vi "init.vi"(8 "error in":errorcluster, 10 "TBM module configuration in":refnum<class "TBM module configuration.lvclass">, 11 "shared memory module runtime":refnum<class "Shared Memory Runtime.lvclass">) -> (0 "error out":errorcluster, 1 "data allocations":T1, 2 "execution settings":T4, 3 "shared memory module runtime out":refnum<class "Shared Memory Runtime.lvclass">)   [LabVIEW 2013, in "Shared Memory Runtime.lvclass"]
doc: "Provides an interface for initializing a module at runtime. While this interface performs no operations, a child should provide an override which may open any necessary references or sessions, allocate necessary memory, and perform any final configuration validataion before providing the full configuration <b>execution data</b> to the calling process.Copyright 2016 National Instruments Corporation\n\nLicensed under the Apache License, Version 2.0 (the \"License\"); you may not use this file except in compliance with the License. You may obtain a copy of the License at http://www.apache.org/licenses/LICENSE-2.0\nUnless required by applicable law or agreed to in writing, software distributed under the License is distributed on an \"AS IS\" BASIS, WITHOUT WARRANTIES OR CONDITIONS OF ANY KIND, either express or implied. See the License for the specific language governing permissions and limitations under the License."
uses:
  Shared Memory Runtime.lvclass
  <vilib>/NI/Tag Bus Module Framework/module configuration/TBM module configuration.lvclass
  <vilib>/NI/Tag Bus Module Framework/runtime/execution settings.ctl
  <vilib>/NI/Tag Bus Module Framework/channel/data tables.ctl
  <vilib>/NI/Tag Bus/dictionary/data dictionary.lvclass
  <vilib>/NI/Tag Bus/dictionary table pair.ctl
  <vilib>/NI/Tag Bus/table/data table.ctl
  configuration/Shared Memory Configuration.lvclass
  configuration/Shared Memory Configuration.lvclass/Shared Memory Configuration.ctl
  configuration/Read lines.vi
  configuration/read read directory.vi
  configuration/read write directory.vi
  <vilib>/NI/Tag Bus Module Framework/channel/TBM channel.lvclass
  <vilib>/NI/Tag Bus Module Framework/runtime/TBM module execution interface.lvclass
  <vilib>/NI/Tag Bus/tag bus.lvlib
  <vilib>/NI/Tag Bus/table/data table.lvlib
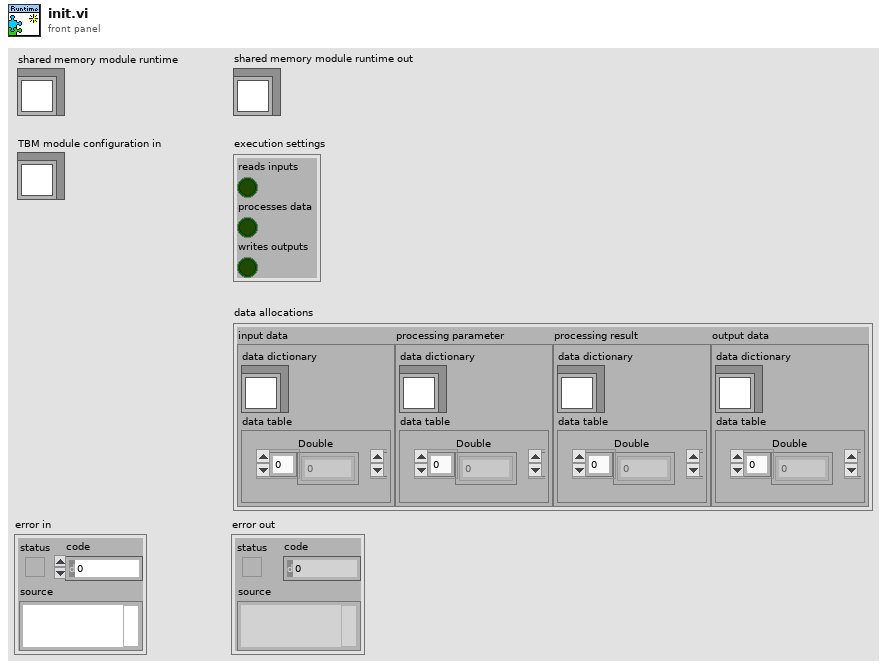
[diagram p1: front panel]
types:
  T1 = typedef "TBM channel.lvclass/data tables.ctl" = cluster{"input data":T2, "processing parameter":T2, "processing result":T2, "output data":T2}
  T2 = typedef "tag bus.lvlib/dictionary table pair.ctl" = cluster{"data dictionary":refnum<class "data dictionary.lvclass">, "data table":T3}
  T3 = typedef "tag bus.lvlib/data table.lvlib/data table.ctl" = cluster{"Double":dbl[], "Single":sgl[], "I64":i64[], "I32":i32[], "I16":i16[], "I8":i8[], "U64":u64[], "U32":u32[], "U16":u16[], "U8":u8[], "Boolean":bool[], "String":string[], "Array of Double":cluster{"DBL Array":dbl[]}[], "Array of Single":cluster{"SGL Array":sgl[]}[], "Array of I64":cluster{"I64 Array":i64[]}[], "Array of I32":cluster{"I32 Array":i32[]}[], "Array of I16":cluster{"I16 Array":i16[]}[], "Array of I8":cluster{"I8 Array":i8[]}[], "Array of U64":cluster{"U64 Array":u64[]}[], "Array of U32":cluster{"U32 Array":u32[]}[], "Array of U16":cluster{"U16 Array":u16[]}[], "Array of U8":cluster{"U8 Array":u8[]}[], "Array of Boolean":cluster{"Boolean Array":bool[]}[], "Array of String":cluster{"String Array":string[]}[]}
  T4 = typedef "TBM module execution interface.lvclass/execution settings.ctl" = cluster{"reads inputs":bool, "processes data":bool, "writes outputs":bool}
  T5 = typedef "Shared Memory Configuration.lvclass/line configuration.ctl" = cluster{"name":string, "data type":T6, "channel":refnum<class "TBM channel.lvclass">}
  T6 = typedef "tag bus.lvlib/tag descriptor.lvclass/Data Type.ctl" = enum16{"Double", "Single", "I64", "I32", "I16", "I8", "U64", "U32", "U16", "U8", "Boolean", "String", "Array of Double", "Array of Single", "Array of I64", "Array of I32", "Array of I16", "Array of I8", "Array of U64", "Array of U32", "Array of U16", "Array of U8", "Array of Boolean", "Array of String"}
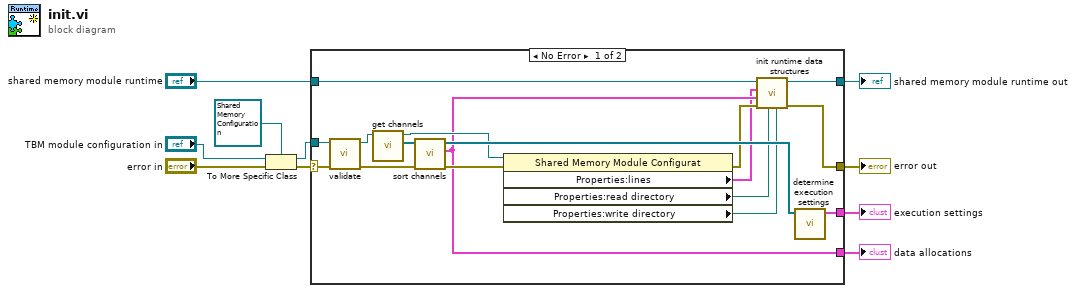
[diagram p0: block diagram]
diagram:
  n1 = To More Specific Class(target class=refnum<class "Shared Memory Configuration.lvclass"> refnum ("Synchronous module configuration"), reference="TBM module configuration in", error in="error in") -> (specific class reference=w9:refnum<class "Shared Memory Configuration.lvclass">, error out=w10:errorcluster)
  n2 = case shown="No Error" w10 {
    selector: w10 -> [w23 w28]
    tunnel: w9 -> [w22 _]
    tunnel: "shared memory module runtime" -> [w16 w29]
    tunnel: [w15 w29] -> w5
    tunnel: [w18 w28] -> w4
    tunnel: [w14 _] -> w2
    tunnel: [w26 _] -> w3
    frame No Error {
      n3 = call-dynamic "validate.vi"("error in"=w23, "shared memory module configuration"=w22) -> ("error out"=w24:errorcluster, "shared memory module configuration out"=w21:refnum<class "Shared Memory Configuration.lvclass">)  [unwired: 8 in]
      n4 = call-dynamic "get channels.vi"("shared memory module configuration"=w21) -> ("channels"=w20:refnum<class "TBM channel.lvclass">[], "shared memory module configuration out"=w19:refnum<class "Shared Memory Configuration.lvclass">)  [unwired: 9 in]
      n5 = call <vilib>:"sort channels.vi"("error in"=w24, "channels in"=w20) -> ("error out"=w27:errorcluster, "data allocations"=w14:T1, "channels out"=w25:refnum<class "TBM channel.lvclass">[])  [unwired: 7 in]
      n6 = property class="Shared Memory Module Configurat"(reference=w19, error in=w27) -> (error out=w17:errorcluster, "Properties:lines"=w13:T5[], "Properties:read directory"=w11:path, "Properties:write directory"=w12:path)  [unwired: 1 out]
      n7 = call "init runtime data structures.vi"("write directory"=w12, "read directory"=w11, "error in"=w17, "data allocations"=w14, "lines"=w13, "shared memory module runtime in"=w16) -> ("error out"=w18:errorcluster, "shared memory module runtime out"=w15:refnum<class "Shared Memory Runtime.lvclass">)  [unwired: 4 in]
      n8 = call <vilib>:"determine execution settings.vi"("channels"=w25) -> ("execution settings"=w26:T4)  [unwired: 10 in]
    }
    frame Error {
    }
  }
  "error out" <- w4
  "shared memory module runtime out" <- w5
  "execution settings" <- w3
  "data allocations" <- w2
